vi "Periodic Tasks.vi"(8 "error in":errorcluster) -> ()   [LabVIEW 2014]
doc: "This VI runs in parallel to other tasks. It can contain as many user-defined periodic loops as you need. These can carry out PID or other sorts of timed response."
uses:
  <vilib>/Rock Robotics/WPI/Joystick/WPI_JoystickGetSetRefNum.vi
  <vilib>/Rock Robotics/WPI/RobotDrive/WPI_RobotDriveGetSetRefNum.vi
panel:
  out "Distance":dbl
  out "Theta (Rad)":dbl
  out "Theta (Deg)":dbl
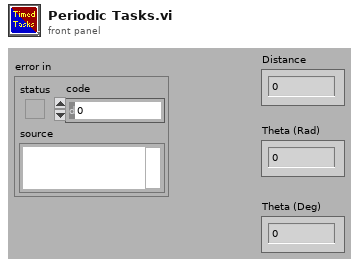
[diagram p1: front panel]
types:
  T1 = typedef "WPI_JoystickDevRef.ctl" = cluster{"Device":T2}
  T2 = typedef "WPI_JoystickDeviceEnum.ctl" = enum16{"USB 0", "USB 1", "USB 2", "USB 3", "USB 4", "USB 5"}
  T3 = typedef "WPI_RobotDriveDevRef.ctl" = cluster{"DevStatus":errorcluster, "Motors[]":T4[], "Square Inputs":bool, "Max Output":dbl}
  T4 = typedef "WPI_MotorControlDeviceRef.ctl" = cluster{"DeviceStatus":errorcluster, "Type":T5, "PWM":cluster{"Controller":T6, "PWM Channel":T7, "DeadBand":T8}, "CAN":cluster{"Device Number":u8, "Control Mode":T9, "Semaphore":T10, "Max Vout":dbl, "TalonSRX Control Mode":T11}, "Invert":bool, "TransformRef":T12, "InvTransformRef":T12}
  T5 = typedef "WPI_MotorControlType.ctl" = enum16{"PWM", "CAN", "CANTalonSRX"}
  T6 = typedef "FPGA_TypedefDigitalModule.ctl" = enum16{"Controller 1"}
  T7 = typedef "FPGA_DIOPWMChannel.ctl" = enum8{"PWM 0", "PWM 1", "PWM 2", "PWM 3", "PWM 4", "PWM 5", "PWM 6", "PWM 7", "PWM 8", "PWM 9", "PWM MXP 0", "PWM MXP 1", "PWM MXP 2", "PWM MXP 3", "PWM MXP 4", "PWM MXP 5", "PWM MXP 6", "PWM MXP 7", "PWM MXP 8", "PWM MXP 9", "Invalid"}
  T8 = typedef "WPI_PWMDeadband.ctl" = cluster{"Name":string, "maxPositivePwm":i32, "minPositivePwm":i32, "centerPwm":i32, "maxNegativePwm":i32, "minNegativePwm":i32, "angularRange":u16}
  T9 = typedef "WPI_CANJaguar_ControlMode.ctl" = enum8{"Percent VBus", "Current", "Speed", "Position", "Voltage"}
  T10 = typedef "Semaphore RefNum" = refnum<k1>
  T11 = typedef "WPI_CANTalonSRX_APIControlMode.ctl" = enum8{"Percent VBus", "Speed", "Position", "Slave", "Unchanged / Invalid"}
  T12 = typedef "WPI_PWMTransform_ConPane.ctl" = refnum<vi>
  T13 = cluster{"JoystickDevRef":T1, "RobotDriveDevRef":T3}
  T14 = cluster{"Axes[0]":dbl, "Axes[1]":dbl, "Axes[2]":dbl, "Axes[3]":dbl, "Axes[4]":dbl, "Axes[5]":dbl, "Axes[6]":dbl, "Axes[7]":dbl, "Axes[8]":dbl}
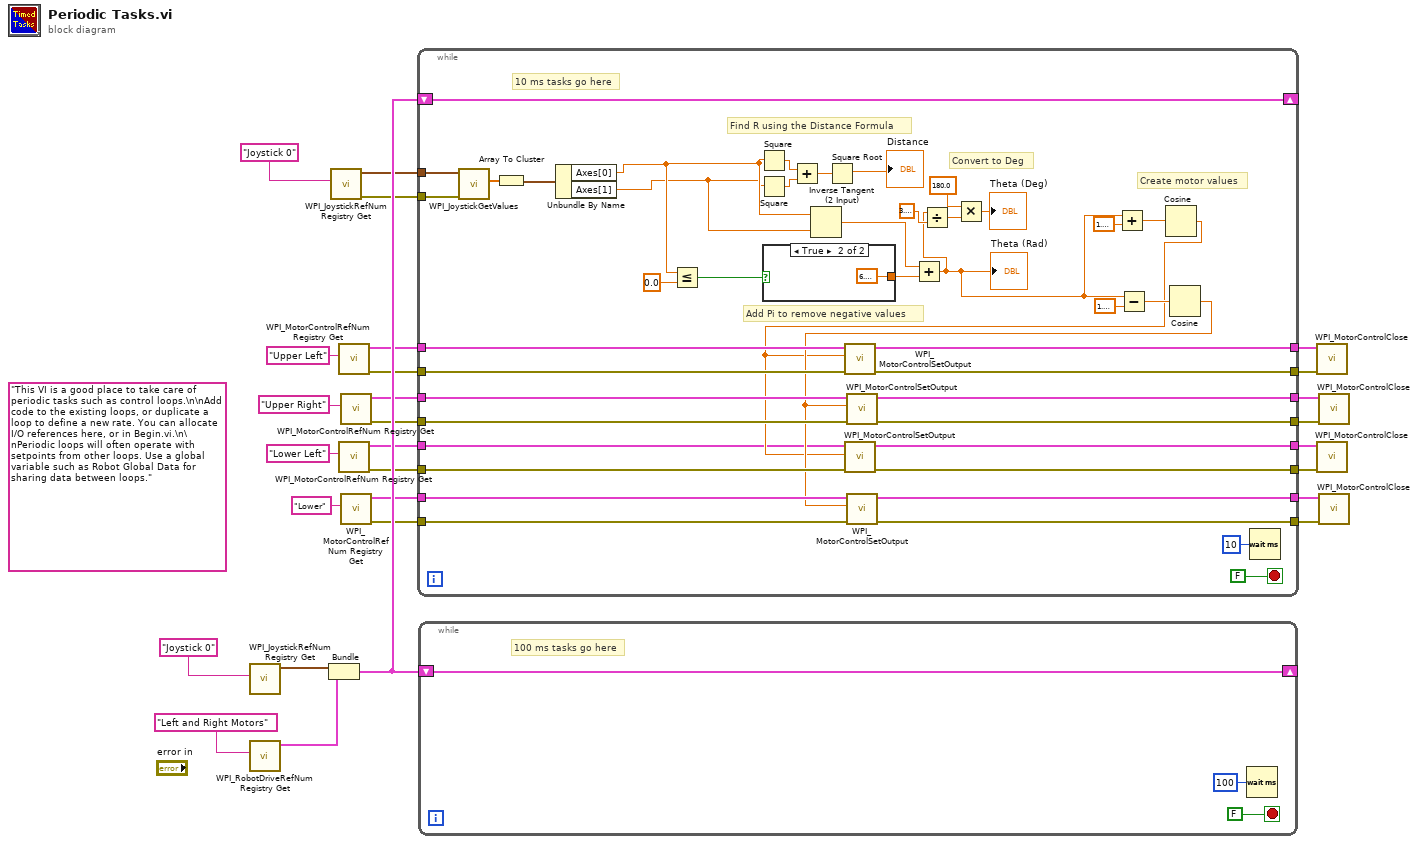
[diagram p0: block diagram]
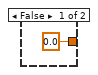
[diagram p2: hidden frame]
diagram:
  (unwired) "This VI is a good place to take care of periodic tasks such as control loops.\n\nAdd code to the existing loops, or duplicate a loop to define a new rate. You can allocate I/O references here, or in Begin.vi.\n\nPeriodic loops will often operate with setpoints from other loops. Use a global variable such as Robot Global Data for sharing data between loops."
  n1 = call <vilib>:"WPI_JoystickRefNum Registry Get.vi"("refnum name"="Joystick 0") -> ("JoystickDevRef"=w26:T1)  [unwired: 1 in, 9 out]
  n2 = call <vilib>:"WPI_RobotDriveRefNum Registry Get.vi"("refnum name"="Left and Right Motors") -> ("RobotDriveDevRef"=w25:T3)  [unwired: 1 in, 9 out]
  n3 = Bundle("JoystickDevRef"=w26, "RobotDriveDevRef"=w25) -> (w24:T13)  [unwired: 1 out]
  n4 = call <vilib>:"WPI_JoystickRefNum Registry Get.vi"("refnum name"="Joystick 0") -> ("error out"=w21:errorcluster, "JoystickDevRef"=w22:T1)  [unwired: 1 in, 8 out]
  n5 = call <vilib>:"WPI_MotorControlRefNum Registry Get.vi"("refnum name"="Upper Left") -> ("error out"=w18:errorcluster, "MotorControlDevRef"=w20:T4)  [unwired: 9 in]
  n6 = call <vilib>:"WPI_MotorControlRefNum Registry Get.vi"("refnum name"="Lower Left") -> ("error out"=w9:errorcluster, "MotorControlDevRef"=w2:T4)  [unwired: 9 in]
  n7 = call <vilib>:"WPI_MotorControlRefNum Registry Get.vi"("refnum name"="Upper Right") -> ("error out"=w10:errorcluster, "MotorControlDevRef"=w13:T4)  [unwired: 9 in]
  n8 = call <vilib>:"WPI_MotorControlRefNum Registry Get.vi"("refnum name"="Lower") -> ("error out"=w4:errorcluster, "MotorControlDevRef"=w7:T4)  [unwired: 9 in]
  n9 = while {
    shift-right: [w70] -> _
    shift-left: w24 -> [w70]
    tunnel: w22 -> [w69]
    tunnel: w21 -> [w68]
    tunnel: w20 -> [w51]
    tunnel: [w50] -> w19
    tunnel: w18 -> [w49]
    tunnel: [w48] -> w17
    tunnel: w13 -> [w47]
    tunnel: [w46] -> w12
    tunnel: [w45] -> w11
    tunnel: w10 -> [w44]
    tunnel: w9 -> [w43]
    tunnel: [w42] -> w8
    tunnel: w7 -> [w41]
    tunnel: [w40] -> w6
    tunnel: [w39] -> w5
    tunnel: w4 -> [w38]
    tunnel: w2 -> [w30]
    tunnel: [w29] -> w1
    stop <- FALSE stop-if-true
    # "Create motor values"
    # "Find R using the Distance Formula"
    # "Add Pi to remove negative values"
    # "Convert to Deg"
    # "10 ms tasks go here"
    n10 = call <vilib>:"WPI_JoystickGetValues.vi"("error in (no error)"=w68, "JoystickDevRef"=w69) -> ("Axes"=w67:dbl[])  [unwired: 5 in, 4 out]
    n11 = Array To Cluster(array=w67) -> (cluster=w66:T14)
    n12 = Unbundle By Name(w66) -> ("Axes[0]"=w53:dbl, "Axes[1]"=w52:dbl)
    n13 = Less Or Equal?(x=w53, y=0.0) -> (x <= y?=w54:bool)
    n14 = Square(x=w53) -> (x^2=w64:dbl)
    n15 = Square(x=w52) -> (x^2=w65:dbl)
    n16 = case shown="True" w54 {
      tunnel: [0.0 6.283185307179586] -> w60
      frame False {
      }
      frame True {
      }
    }
    n17 = Add(x=w64, y=w65) -> (x+y=w63:dbl)
    n18 = Inverse Tangent (2 Input)(1:w52, 2:w53) -> (0:w56:dbl)
    n19 = Square Root(x=w63) -> (sqrt(x)=→"Distance":dbl)
    n20 = Add(x=w56, y=w60) -> (x+y=w35:dbl)
    "Theta (Rad)" <- w35
    n21 = Divide(x=w35, y=3.141592653589793) -> (x/y=w59:dbl)
    n22 = Multiply(x=180.0, y=w59) -> (x*y=→"Theta (Deg)":dbl)
    n23 = Add(x=w35, y=1.5707963267948966) -> (x+y=w34:dbl)
    n24 = Subtract(x=w35, y=1.5707963267948966) -> (x-y=w33:dbl)
    n25 = Cosine(x=w34) -> (cos(x)=w31:dbl)
    n26 = call <vilib>:"WPI_MotorControlSetOutput.vi"("error in (no error)"=w49, "Output"=w31, "MotorControlDevRef"=w51) -> ("error out"=w48:errorcluster, "MotorControlDevRef"=w50:T4)  [unwired: 6 in, 1 out]
    n27 = call <vilib>:"WPI_MotorControlSetOutput.vi"("error in (no error)"=w43, "Output"=w31, "MotorControlDevRef"=w30) -> ("error out"=w42:errorcluster, "MotorControlDevRef"=w29:T4)  [unwired: 6 in, 1 out]
    n28 = Cosine(x=w33) -> (cos(x)=w32:dbl)
    n29 = call <vilib>:"WPI_MotorControlSetOutput.vi"("error in (no error)"=w44, "Output"=w32, "MotorControlDevRef"=w47) -> ("error out"=w45:errorcluster, "MotorControlDevRef"=w46:T4)  [unwired: 6 in, 1 out]
    n30 = call <vilib>:"WPI_MotorControlSetOutput.vi"("error in (no error)"=w38, "Output"=w32, "MotorControlDevRef"=w41) -> ("error out"=w39:errorcluster, "MotorControlDevRef"=w40:T4)  [unwired: 6 in, 1 out]
    n31 = Wait (ms)(milliseconds to wait=u32 10) -> ()  [unwired: 1 out]
  }
  n32 = while {
    shift-right: [w75] -> _
    shift-left: w24 -> [w75]
    stop <- FALSE stop-if-true
    # "100 ms tasks go here"
    n33 = Wait (ms)(milliseconds to wait=u32 100) -> ()  [unwired: 1 out]
  }
  n34 = call <vilib>:"WPI_MotorControlClose.vi"("error in (no error)"=w17, "MotorControlDevRef"=w19) -> ()  [unwired: 9 in, 1 out]
  n35 = call <vilib>:"WPI_MotorControlClose.vi"("error in (no error)"=w8, "MotorControlDevRef"=w1) -> ()  [unwired: 9 in, 1 out]
  n36 = call <vilib>:"WPI_MotorControlClose.vi"("error in (no error)"=w11, "MotorControlDevRef"=w12) -> ()  [unwired: 9 in, 1 out]
  n37 = call <vilib>:"WPI_MotorControlClose.vi"("error in (no error)"=w5, "MotorControlDevRef"=w6) -> ()  [unwired: 9 in, 1 out]
